vi "OpenCreateReplace Dataset.vi"(5 "operation (open or create)":T1=enum."open or create", 6 "HDF5 Property List Ref":T2, 7 "Dataset Path":string, 8 "error in (no error)":errorcluster, 9 "HDF5 Dataspace Ref":T2, 10 "HDF5 Datatype Ref":T2, 11 "HDF5 Ref":T2) -> (0 "error out":errorcluster, 2 "HDF5 Dataset Ref":T2, 3 "HDF5 Ref out":T2)   [LabVIEW 2017]
doc: "Opens, creates or replaces an dataset."
uses:
  <vilib>/UPVI/lvhdf5/library.llb/HDF5 Ref.ctl
  <vilib>/UPVI/lvhdf5/dataset.llb/LVH5D Operation.ctl
  <vilib>/UPVI/lvhdf5/group.llb/OpenCreateGroup (Array).vi
panel:
  # "LVHDF5 Toolkit\nCopyright (c) 2005-2013 by Jason D. Sommerville\nCopyright (c) 2014 by UPVI, LLC.\n\nThis use and distribution of this file is governed by the terms found in \nLICENSE.txt distributed with this toolkit and installed at\n <user.lib>\\_lvhdf5\\LICENSE.txt"
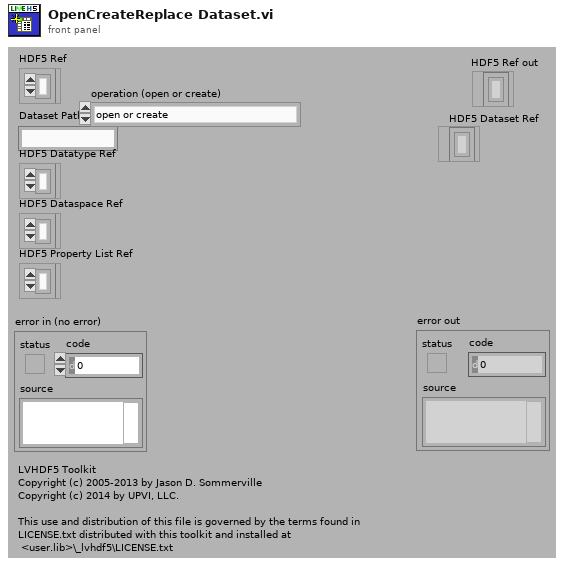
[diagram p1: front panel]
types:
  T1 = typedef "LVH5D Operation.ctl" = enum16{"open", "replace", "create", "open or create", "create or replace", "create or replace with confirmation"}
  T2 = typedef "HDF5 Ref.ctl" = refnum<k1>
  T3 = enum16{"Left Button", "Center Button", "Right Button", "Window Close"}
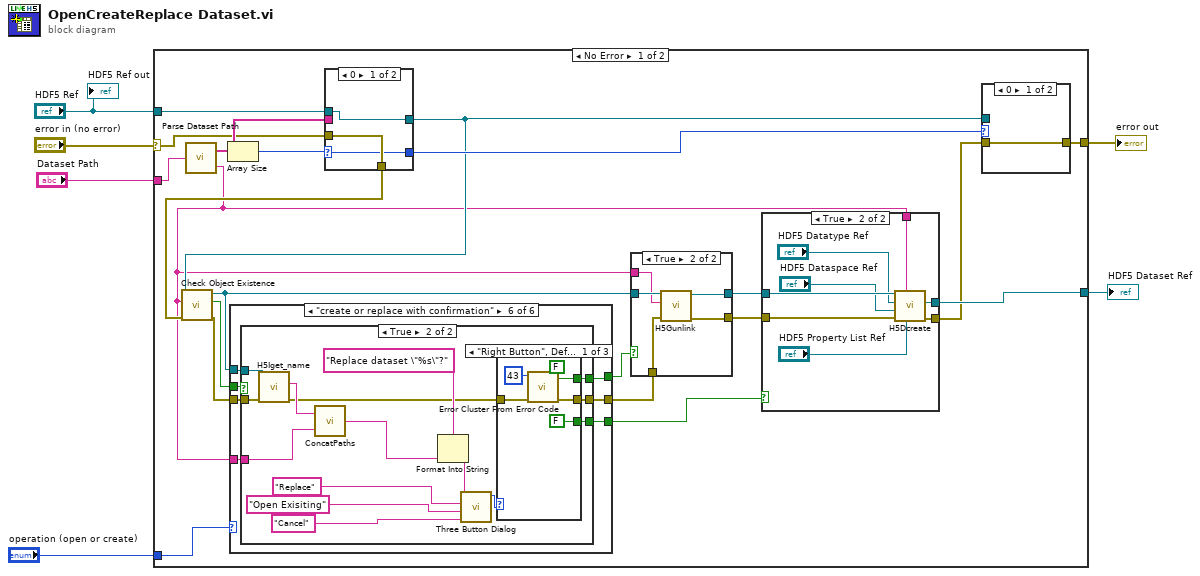
[diagram p0: block diagram]
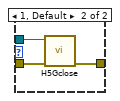
[diagram p2: hidden frame]
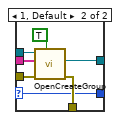
[diagram p3: hidden frame]
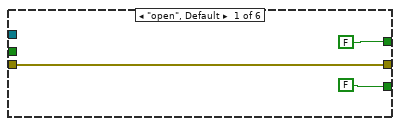
[diagram p4: hidden frame]
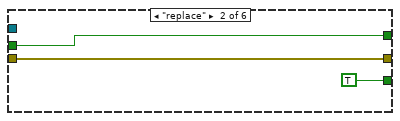
[diagram p5: hidden frame]
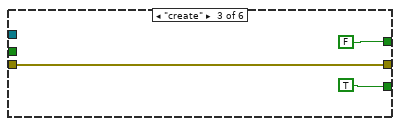
[diagram p6: hidden frame]
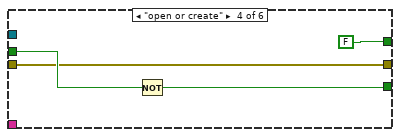
[diagram p7: hidden frame]
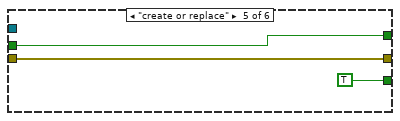
[diagram p8: hidden frame]
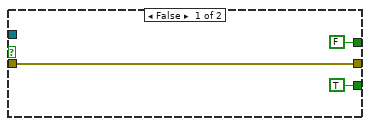
[diagram p9: hidden frame]
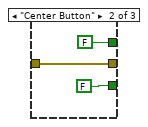
[diagram p10: hidden frame]
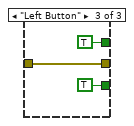
[diagram p11: hidden frame]
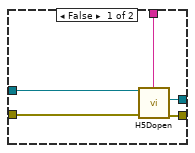
[diagram p13: hidden frame]
diagram:
  n1 = case shown="No Error" "error in (no error)" {
    selector: "error in (no error)" -> [w8 w114]
    tunnel: [w10 w114] -> w5
    tunnel: "HDF5 Ref" -> [w15 _]
    tunnel: "operation (open or create)" -> [w25 _]
    tunnel: "Dataset Path" -> [w14 _]
    tunnel: [w12 _] -> w2
    frame No Error {
      n2 = call <vilib>:"Parse Dataset Path.vi"("Dataset path"=w14) -> ("Groups"=w18:string[], "Dataset"=w7:string)
      n3 = Array Size(array=w18) -> (size(s)=w17:i32)
      n4 = case shown="0" w17 {
        selector: w17 -> [w32 w36]
        tunnel: w15 -> [w33 w41]
        tunnel: w18 -> [_ w40]
        tunnel: [w33 w39] -> w13
        tunnel: w8 -> [w34 w38]
        tunnel: [w34 w37] -> w9
        tunnel: [w32 w36] -> w16
        frame 0 {
        }
        frame 1, Default {
          n5 = call-poly <vilib>:"OpenCreateGroup.vi"("Create if not found (F)"=TRUE, "error in (no error)"=w38, "Array of Groups"=w40, "HDF5 Ref"=w41) -> ("error out"=w37:errorcluster, "HDF5 Group Ref"=w39:T2)  [unwired: 5 in, 1 out]
        }
      }
      n6 = call <vilib>:"Check Object Existence.vi"("error in (no error)"=w9, "name"=w7, "HDF5 Ref"=w13) -> ("error out"=w21:errorcluster, "Exists"=w20:bool, "HDF5 Ref out"=w22:T2)  [unwired: 4 in]
      n7 = case shown="\"create or replace with confirmation\"" w25 {
        tunnel: w20 -> [_ w47 _ w53 w56 w59]
        tunnel: [FALSE TRUE TRUE w52 TRUE w64] -> w24
        tunnel: [FALSE w47 FALSE FALSE w56 w61] -> w23
        tunnel: w22 -> [_ _ _ _ _ w63]
        tunnel: w21 -> [w42 w45 w48 w51 w55 w62]
        tunnel: [w42 w45 w48 w51 w55 w60] -> w19
        tunnel: w7 -> [_ _ _ _ _ w58]
        frame "open", Default {
        }
        frame "replace" {
        }
        frame "create" {
        }
        frame "open or create" {
          n8 = Not(x=w53) -> (.not. x?=w52:bool)
        }
        frame "create or replace" {
        }
        frame "create or replace with confirmation" {
          n9 = case shown="True" w59 {
            tunnel: [TRUE w82] -> w64
            tunnel: w63 -> [_ w81]
            tunnel: w62 -> [w65 w80]
            tunnel: [FALSE w76] -> w61
            tunnel: [w65 w75] -> w60
            tunnel: w58 -> [_ w70]
            frame False {
            }
            frame True {
              n10 = call <vilib>:"H5Iget_name.vi"("error in (no error)"=w80, "HDF5 Ref"=w81) -> ("error out"=w68:errorcluster, "Name"=w71:string)  [unwired: 4 in, 2 out]
              n11 = call <vilib>:"ConcatPaths.vi"("Path2"=w70, "Path1"=w71) -> ("Path1/Path2"=w69:string)
              n12 = Format Into String(format string="Replace dataset \"%s\"?" ("message"), w69) -> (resulting string=w78:string)  [unwired: 2 in, 1 out]
              n13 = call <vilib>:"Three Button Dialog.vi"("Right Button Text (\"Cancel\")"="Cancel" ("Right Button Text (\"Cancel\")"), "Center Button Text (\"No\")"="Open Exisiting" ("F button name (\"Cancel\")"), "Left Button Text (\"Yes\")"="Replace" ("T button name (\"OK\")"), "message"=w78) -> ("Which Button?"=w77:T3)  [unwired: 7 in]
              n14 = case shown="\"Right Button\", Default" w77 {
                tunnel: [FALSE FALSE TRUE] -> w82
                tunnel: [FALSE FALSE TRUE] -> w76
                tunnel: w68 -> [w87 w88 w93]
                tunnel: [w85 w88 w93] -> w75
                frame "Right Button", Default {
                  n15 = call <vilib>:"Error Cluster From Error Code.vi"("error in (no error)"=w87, "error code (0)"=43) -> ("error out"=w85:errorcluster)  [unwired: 7 in]
                }
                frame "Center Button" {
                }
                frame "Left Button" {
                }
              }
            }
          }
        }
      }
      n16 = case shown="True" w23 {
        tunnel: w22 -> [w95 w100]
        tunnel: w7 -> [_ w99]
        tunnel: [w95 w98] -> w26
        tunnel: [w94 w97] -> w27
        tunnel: w19 -> [w94 w96]
        frame False {
        }
        frame True {
          n17 = call <vilib>:"H5Gunlink.vi"("error in (no error)"=w96, "Name"=w99, "HDF5 Ref"=w100) -> ("error out"=w97:errorcluster, "HDF5 Ref out"=w98:T2)  [unwired: 5 in]
        }
      }
      n18 = case shown="True" w24 {
        tunnel: w27 -> [w101 w113]
        tunnel: w26 -> [w103 w112]
        tunnel: w7 -> [w102 w111]
        tunnel: [w104 w107] -> w12
        tunnel: [w105 w106] -> w11
        frame False {
          n19 = call <vilib>:"H5Dopen.vi"("error in (no error)"=w101, "name"=w102, "HDF5 Ref"=w103) -> ("error out"=w105:errorcluster, "HDF5 Dataset Ref"=w104:T2)  [unwired: 4 in, 1 out]
        }
        frame True {
          n20 = call <vilib>:"H5Dcreate.vi"("Dataset Creation Property List"="HDF5 Property List Ref", "Name"=w111, "error in (no error)"=w113, "HDF5 Dataspace Ref"="HDF5 Dataspace Ref", "HDF5 Datatype Ref"="HDF5 Datatype Ref", "HDF5 Location Ref"=w112) -> ("error out"=w106:errorcluster, "HDF5 Dataset Ref"=w107:T2)  [unwired: 3 in, 1 out]
        }
      }
      n21 = case shown="0" w16 {
        tunnel: w13 -> [_ w31]
        tunnel: w11 -> [w28 w30]
        tunnel: [w28 w29] -> w10
        frame 0 {
        }
        frame 1, Default {
          n22 = call <vilib>:"H5Gclose.vi"("error in (no error)"=w30, "HDF5 Group Ref"=w31) -> ("error out"=w29:errorcluster)  [unwired: 7 in]
        }
      }
    }
    frame Error {
    }
  }
  "error out" <- w5
  "HDF5 Dataset Ref" <- w2
  "HDF5 Ref out" <- "HDF5 Ref"
